vi "Goal_Clamp_on_Move.vi"(5 "Goal Down":u8=193, 7 "Goal Up":u8=70, 8 "Law Down":u8=6, 9 "Law Up":u8=201, 10 "Numeric":i32, 11 "60 Goal?":bool) -> ()   [LabVIEW 2012, in "Serenity_mk2.lvrbt"]
uses:
  Serenity_mk2.lvrbt
  <vilib>/NXT/Hardware/Plugins/Tetrix 180 deg Servo/Tetrix180ServoAddress.ctl
  <vilib>/NXT/Hardware/Plugins/Tetrix DC Motor/TetrixDCMotorAddress.ctl
  <vilib>/NXT/NXTIO Xnodes/NXTIONodeSubVIs/TETRIX IO Move Servos.vi
  <vilib>/NXT/NXTIO Xnodes/NXTIONodeSubVIs/TETRIX IO Move DC Motors.vi
  <vilib>/NXT/Subs/LVHSConnector.ctl
  <vilib>/NXT/NXTIO Xnodes/AddressXNode/NXTIOAddress.xnode
  <vilib>/NXT/NXTIO Xnodes/NXTIOXNode/NXTIO.xnode
  <vilib>/NXT/LegoClasses/BrickReference/BrickReference.lvclass
panel:
  in  "Goal Down 2":u8=193
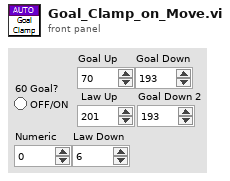
[diagram p1: front panel]
types:
  T1 = typedef "Tetrix180ServoAddress.ctl" = i32
  T2 = typedef "TetrixDCMotorAddress.ctl" = i32
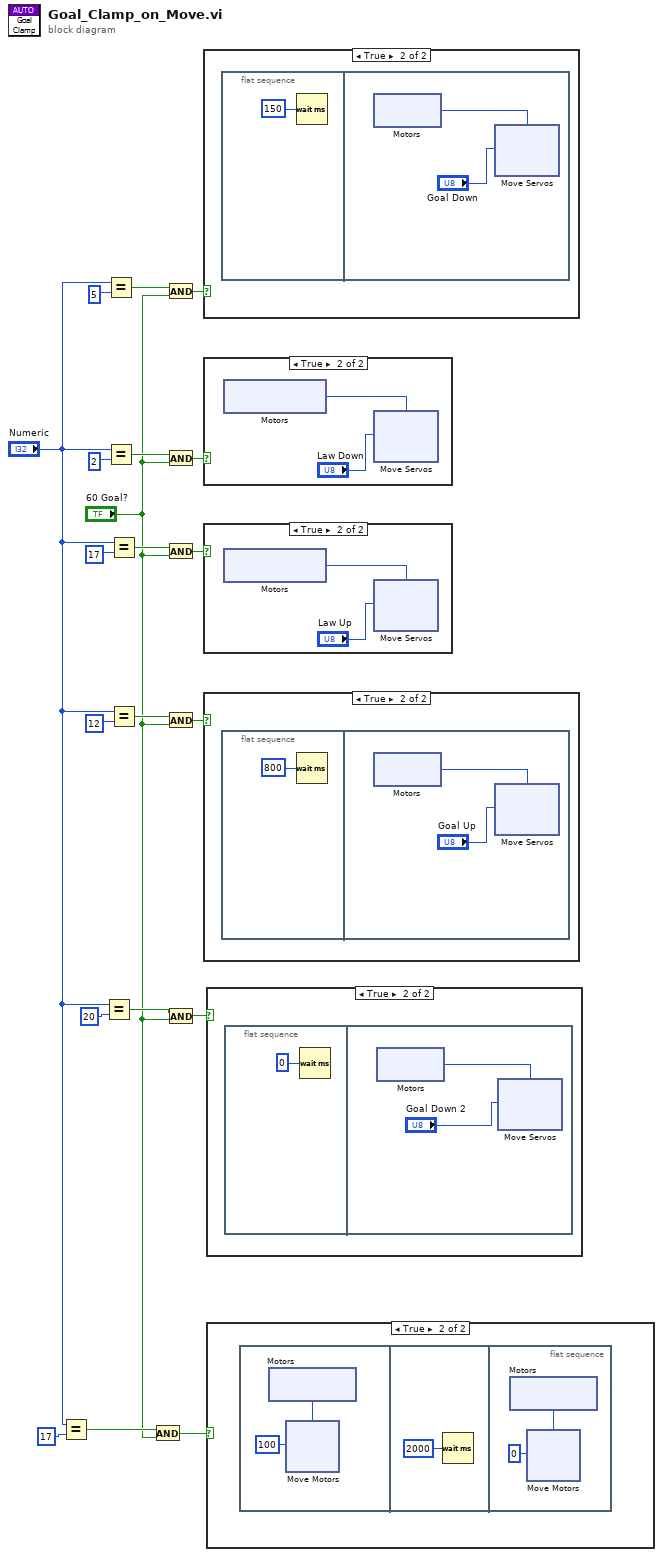
[diagram p0: block diagram]
diagram:
  n1 = Equal?(x="Numeric", y=17) -> (x = y?=w5:bool)
  n2 = Equal?(x="Numeric", y=20) -> (x = y?=w7:bool)
  n3 = Equal?(x="Numeric", y=5) -> (x = y?=w17:bool)
  n4 = Equal?(x="Numeric", y=2) -> (x = y?=w12:bool)
  n5 = Equal?(x="Numeric", y=17) -> (x = y?=w10:bool)
  n6 = Equal?(x="Numeric", y=12) -> (x = y?=w19:bool)
  n7 = And(x=w5, y="60 Goal?") -> (x .and. y?=w1:bool)
  n8 = And(x=w17, y="60 Goal?") -> (x .and. y?=w18:bool)
  n9 = And(x=w12, y="60 Goal?") -> (x .and. y?=w14:bool)
  n10 = And(x=w10, y="60 Goal?") -> (x .and. y?=w9:bool)
  n11 = And(x=w19, y="60 Goal?") -> (x .and. y?=w20:bool)
  n12 = And(x=w7, y="60 Goal?") -> (x .and. y?=w8:bool)
  n13 = case shown="True" w18 {
    frame False {
    }
    frame True {
      n14 = flat-sequence {
        frame #0 {
          n15 = Wait (ms)(milliseconds to wait=u32 150 ("Time (1 sec)")) -> ()  [unwired: 1 out]
        }
        frame #1 {
          n16 = xnode "Motors"() -> ("Motor"=w23:T1)
          n17 = xnode "Move Servos"("Position 1"="Goal Down", "Motors"=w23) -> ()  [unwired: 1 in, 1 out]
        }
      }
    }
  }
  n18 = case shown="True" w14 {
    frame False {
    }
    frame True {
      n19 = xnode "Motors"() -> ("Motor"=w33:T1)
      n20 = xnode "Move Servos"("Position 1"="Law Down", "Motors"=w33) -> ()  [unwired: 1 in, 1 out]
    }
  }
  n21 = case shown="True" w9 {
    frame False {
    }
    frame True {
      n22 = xnode "Motors"() -> ("Motor"=w43:T1)
      n23 = xnode "Move Servos"("Position 1"="Law Up", "Motors"=w43) -> ()  [unwired: 1 in, 1 out]
    }
  }
  n24 = case shown="True" w20 {
    frame False {
    }
    frame True {
      n25 = flat-sequence {
        frame #0 {
          n26 = Wait (ms)(milliseconds to wait=u32 800 ("Time (1 sec)")) -> ()  [unwired: 1 out]
        }
        frame #1 {
          n27 = xnode "Motors"() -> ("Motor"=w53:T1)
          n28 = xnode "Move Servos"("Position 1"="Goal Up", "Motors"=w53) -> ()  [unwired: 1 in, 1 out]
        }
      }
    }
  }
  n29 = case shown="True" w8 {
    frame False {
    }
    frame True {
      n30 = flat-sequence {
        frame #0 {
          n31 = Wait (ms)(milliseconds to wait=u32 0 ("Time (1 sec)")) -> ()  [unwired: 1 out]
        }
        frame #1 {
          n32 = xnode "Motors"() -> ("Motor"=w65:T1)
          n33 = xnode "Move Servos"("Position 1"="Goal Down 2", "Motors"=w65) -> ()  [unwired: 1 in, 1 out]
        }
      }
    }
  }
  n34 = case shown="True" w1 {
    frame False {
    }
    frame True {
      n35 = flat-sequence {
        frame #0 {
          n36 = xnode "Motors"() -> ("Motor"=w75:T2)
          n37 = xnode "Move Motors"("Power/Speed 1"=i8 100, "Motors"=w75) -> ()  [unwired: 1 in, 1 out]
        }
        frame #1 {
          n38 = Wait (ms)(milliseconds to wait=u32 2000) -> ()  [unwired: 1 out]
        }
        frame #2 {
          n39 = xnode "Motors"() -> ("Motor"=w86:T2)
          n40 = xnode "Move Motors"("Power/Speed 1"=i8 0, "Motors"=w86) -> ()  [unwired: 1 in, 1 out]
        }
      }
    }
  }
